vi "Pull Controls Value to DPs.vi"   [LabVIEW 2017, in "TagDB RefManager.lvlib"]
uses:
  TagDB RefManager.lvlib
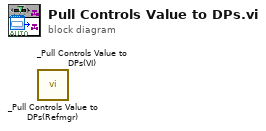
[diagram p0: block diagram]
diagram:
  n1 = call "_Pull Controls Value to DPs(Refmgr).vi"() -> ()  [unwired: 9 in, 3 out]
  n2 = call "_Pull Controls Value to DPs(VI).vi"() -> ()  [unwired: 9 in, 3 out]
